vi "Uso Elapsetime-1.vi"() -> ()   [LabVIEW 2020]
panel:
  out "y":dbl
  in  "stop":bool
  out "Elapsed Time (s)":dbl
  out "Time has Elapsed":bool
  in  "Time Target (s)":dbl=10.0
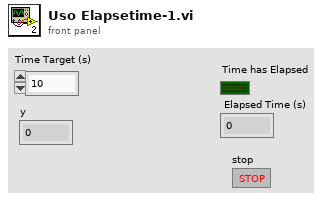
[diagram p1: front panel]
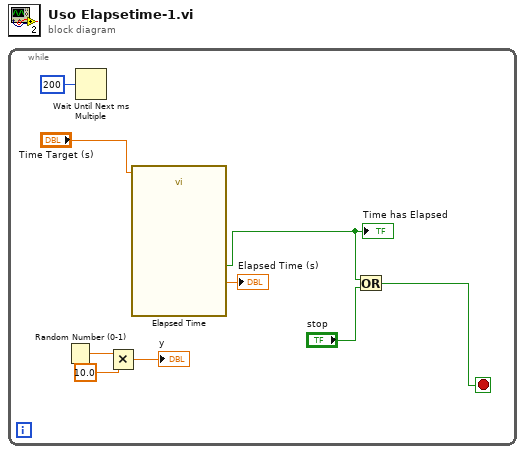
[diagram p0: block diagram]
diagram:
  n1 = while {
    stop <- w1 stop-if-true
    n2 = Random Number (0-1)() -> (number: 0 to 1=w6:dbl)
    n3 = Wait Until Next ms Multiple(millisecond multiple=u32 200) -> ()  [unwired: 1 out]
    n4 = Multiply(x=w6, y=10.0) -> (x*y=→"y":dbl)
    n5 = call "Elapsed Time"("Time Target (s)"="Time Target (s)") -> ("Elapsed Time (s)"=→"Elapsed Time (s)":dbl, "Time has Elapsed"=w3:bool)  [unwired: 11 in, 6 out]
    "Time has Elapsed" <- w3
    n6 = Or(x=w3, y="stop") -> (x .or. y?=w1:bool)
  }
